vi "Close Panel.vi"(8 "error in (no error)":errorcluster, 11 "Panel in":refnum<class "Panel.lvclass">) -> (0 "error out":errorcluster, 3 "Panel out":refnum<class "Panel.lvclass">)   [LabVIEW 2018, in "OOPanel.lvlib" / "Panel.lvclass"]
uses:
  Panel.lvclass
  Panel.lvclass/Panel.ctl
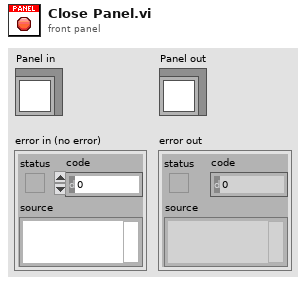
[diagram p1: front panel]
types:
  T1 = typedef "OOPanel.lvlib/Panel.lvclass/Ref Data.ctl" = cluster{"Panel VI":refnum<vi>, "Close":bool, "Panel Events":T2, "Running":bool, "Desired Size":T3, "Subpanel":refnum<vi>, "State":T4}
  T2 = typedef "OOPanel.lvlib/Panel.lvclass/Panel Events.ctl" = cluster{"Close":refnum<user-event>, "Visibility Changed":refnum<user-event>}
  T3 = typedef "OOPanel.lvlib/Panel.lvclass/Desired Size.ctl" = cluster{"Width":i16, "Height":i16}
  T4 = typedef "OOPanel.lvlib/Panel.lvclass/State.ctl" = enum16{"Idle", "Hidden", "Visible", "Subpanel"}
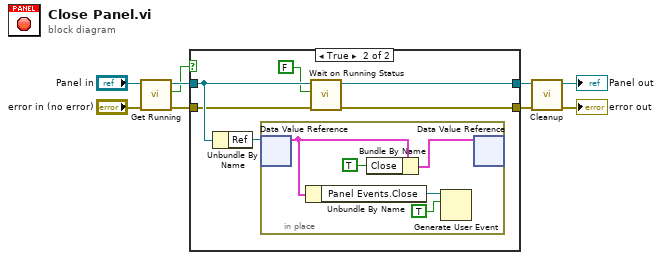
[diagram p0: block diagram]
diagram:
  n1 = call "Get Running.vi"("error in (no error)"="error in (no error)", "Panel in"="Panel in") -> ("error out"=w7:errorcluster, "Running"=w5:bool, "Panel out"=w8:refnum<class "Panel.lvclass">)  [unwired: 7 in]
  n2 = case shown="True" w5 {
    tunnel: w8 -> [w11 w16]
    tunnel: w7 -> [w10 w15]
    tunnel: [w11 w13] -> w4
    tunnel: [w10 w12] -> w3
    frame False {
    }
    frame True {
      n3 = Unbundle By Name(w16) -> ("Ref"=w17:refnum<data-value>)
      n4 = in-place {
        n5 = in-place-dvr #1(w17) -> (w21:T1)  [unwired: 1 out]
        n6 = Unbundle By Name(w21) -> ("Panel Events.Close"=w20:refnum<user-event>)
        n7 = Bundle By Name(cluster=w21, "Close"=TRUE) -> (w19:T1)
        n8 = Generate User Event(user event=w20, event data cluster=TRUE ("event data")) -> ()  [unwired: 2 in, 2 out]
        n9 = in-place-dvr #1(w19) -> ()  [unwired: 2 out]
      }
      n10 = call "Wait on Running Status.vi"("error in (no error)"=w15, "State"=FALSE, "Panel in"=w16) -> ("error out"=w12:errorcluster, "Panel out"=w13:refnum<class "Panel.lvclass">)  [unwired: 7 in]
    }
  }
  n11 = call-dynamic "Cleanup.vi"("error in (no error)"=w3, "Panel in"=w4) -> ("error out"=→"error out":errorcluster, "Panel out"=→"Panel out":refnum<class "Panel.lvclass">)  [unwired: 8 in]
